vi "precess.vi"(2 "Eq2":dbl format="%.4g", 3 "Eq1":dbl format="%.4g", 4 "DEC 1":dbl format="%.10g", 5 "RA 1":dbl format="%.10g") -> (0 "DEC 2":dbl format="%.10g", 1 "RA 2":dbl format="%.10g")   [LabVIEW 2019]
panel:
  out "dec_rad":dbl
  out "ra_rad":dbl
  out "cos(dec)":dbl format="%.6g"
  out "r*x":dbl[](array[numeric]) format="%#_10g"
  out "x":dbl[](array[numeric]) format="%.10g"
  out "r":dbl[](array[numeric]) format="%.10g"
  out "DEC_str":string
  out "RA_str":string
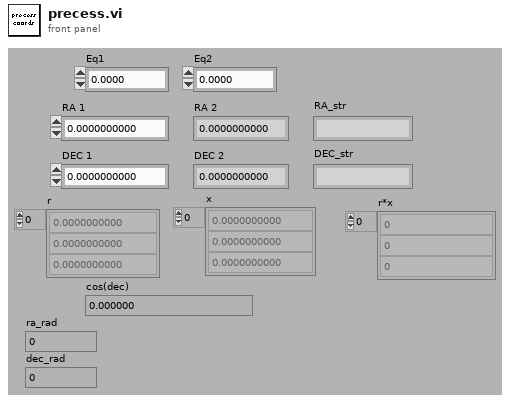
[diagram p1: front panel]
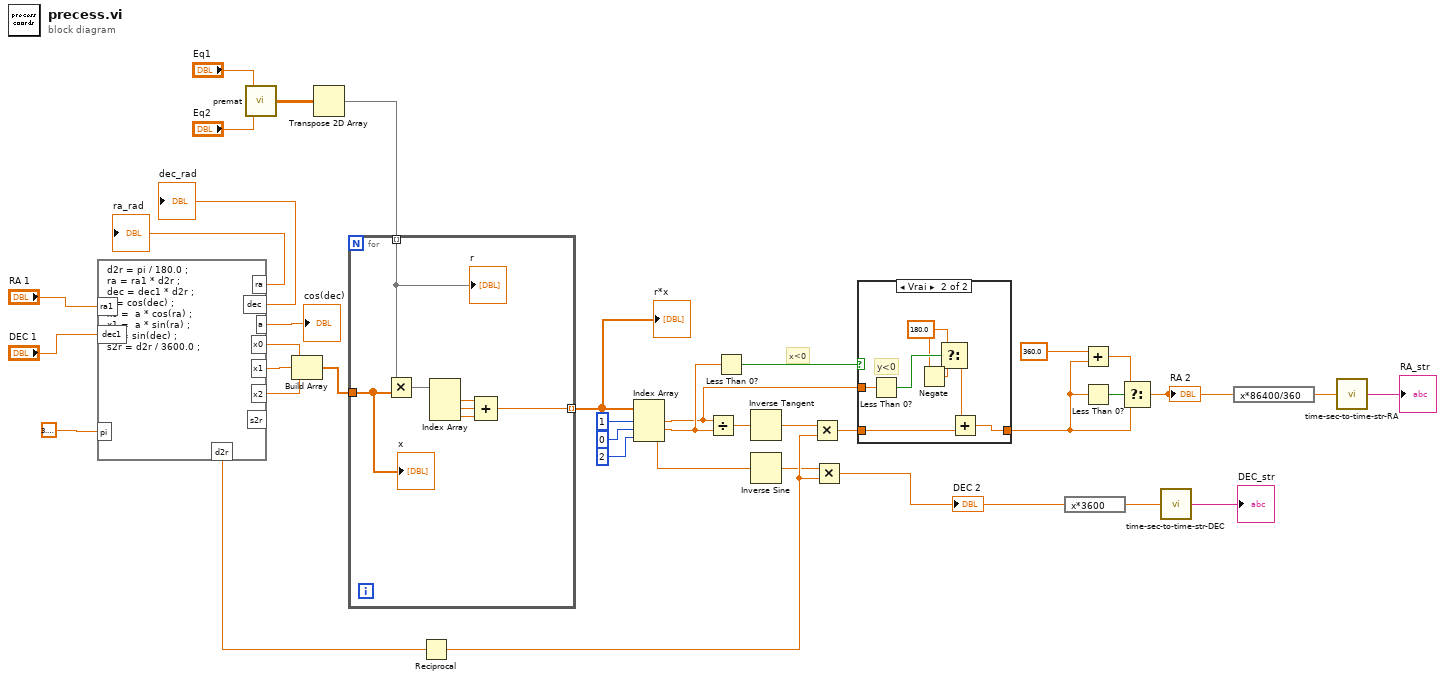
[diagram p0: block diagram]
diagram:
  # "x<0"
  n1 = formula code="d2r = pi / 180.0 ;\nra = ra1 * d2r ;\ndec = dec1 * d2r ;\na = cos(dec) ;\nx0 =  a * cos(ra) ;\nx1 =  a * sin(ra) ;\nx2 = sin(dec) ;\ns2r = d2r / 3600.0 ;"("pi"=3.141592653589793, "ra1"="RA 1", "dec1"="DEC 1") -> ("d2r"=w31:dbl, "ra"=→"ra_rad":dbl, "dec"=→"dec_rad":dbl, "a"=→"cos(dec)":dbl, "x0"=w22:dbl, "x2"=w21:dbl, "x1"=w20:dbl)  [unwired: 1 out]
  n2 = call "premat.vi"("Eq2"="Eq2", "Eq1"="Eq1") -> ("Premat"=w32:dbl[][])
  n3 = Build Array(w22, w20, w21) -> (w33:dbl[])
  n4 = Transpose 2D Array(2D array=w32) -> (transposed array=w13:dbl[][])
  n5 = for {
    tunnel: w33 -> [w45]
    tunnel: w13 -> [w44] mode=indexing
    tunnel: [w39] -> w12 mode=indexing
    n6 = Multiply(x=w44, y=w45) -> (x*y=w43:dbl[])
    n7 = Index Array(array=w43) -> (element #1=w40:dbl, element #2=w41:dbl, element #3=w42:dbl)  [unwired: 3 in]
    n8 = Compound Arithmetic op=ADD(w40, w41, w42) -> (w39:dbl)
    "r" <- w44
    "x" <- w45
  }
  "r*x" <- w12
  n9 = Reciprocal(x=w31) -> (1/x=w30:dbl)
  n10 = Index Array(array=w12, index #1=1 ("index"), index #2=0 ("index"), index #3=2 ("index")) -> (element #1=w1:dbl, element #2=w5:dbl, element #3=w23:dbl)
  n11 = Divide(x=w1, y=w5) -> (x/y=w26:dbl)
  n12 = Less Than 0?(x=w5) -> (x < 0?=w3:bool)
  n13 = Inverse Tangent(1:w26) -> (0:w25:dbl)
  n14 = Inverse Sine(1:w23) -> (0:w24:dbl)
  n15 = Multiply(x=w25, y=w30) -> (x*y=w4:dbl)
  n16 = Multiply(x=w24, y=w30) -> (x*y=w17:dbl)
  "DEC 2" <- w17
  n17 = case shown="Vrai" w3 {
    tunnel: w4 -> [w46 w51]
    tunnel: [w46 w50] -> w2
    tunnel: w1 -> [_ w53]
    frame False {
    }
    frame True {
      w47 = 180.0
      # "y<0"
      n18 = Less Than 0?(x=w53) -> (x < 0?=w52:bool)
      n19 = Negate(x=w47) -> (-x=w48:dbl)
      n20 = Select(t=w47, s=w52, f=w48) -> (s? t:f=w49:dbl)
      n21 = Add(x=w49, y=w51) -> (x+y=w50:dbl)
    }
  }
  n22 = expression code="x*3600"(w17) -> (w15:dbl)
  n23 = Add(x=360.0, y=w2) -> (x+y=w9:dbl)
  n24 = Less Than 0?(x=w2) -> (x < 0?=w10:bool)
  n25 = Select(t=w9, s=w10, f=w2) -> (s? t:f=w11:dbl)
  "RA 2" <- w11
  n26 = call "time-sec-to-time-str-DEC.vi"("Numeric"=w15) -> ("formatted-str"=→"DEC_str":string)
  n27 = expression code="x*86400/360"(w11) -> (w19:dbl)
  n28 = call "time-sec-to-time-str-RA.vi"("Numeric"=w19) -> ("formatted-str"=→"RA_str":string)
